vi "Inject Optitrack Position.vi"() -> (5 "Plug in titles":string[](array[string]), 7 "Plug in values":string[](array[string]))   [LabVIEW 2021]
uses:
  Controls/Post_Process.ctl
  Controls/Setup.ctl
  Globals/Meas_global.vi
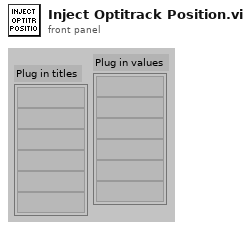
[diagram p1: front panel]
types:
  T1 = typedef "Setup.ctl" = enum16{"Run Program", "Show Setup", "Save Current Setup", "Setup Front Panel"}
  T2 = typedef "Post_Process.ctl" = enum16{"Take New Data", "Post Process Raw Data File"}
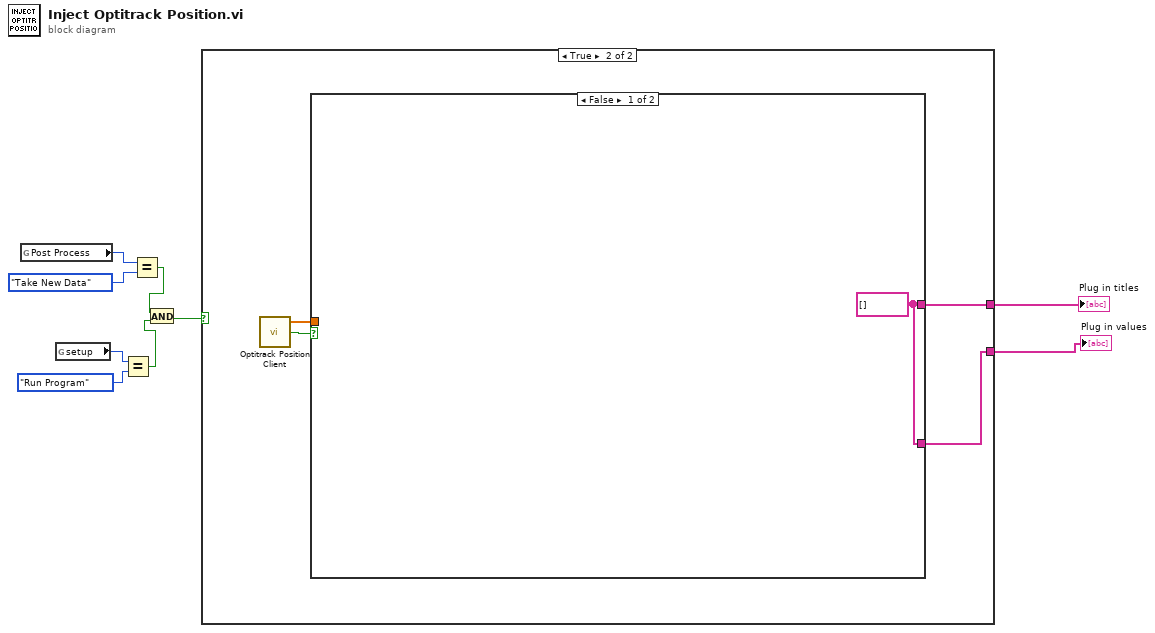
[diagram p0: block diagram]
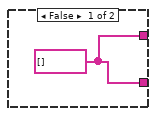
[diagram p2: hidden frame]
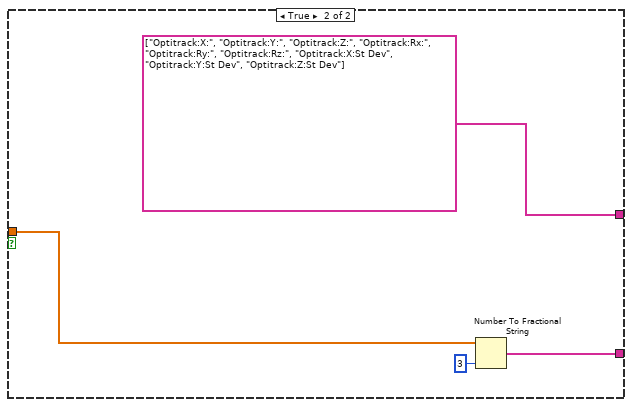
[diagram p3: hidden frame]
diagram:
  n1 = global read "Meas_global.vi" "Post Process"() -> (w4:T2)
  n2 = global read "Meas_global.vi" "setup"() -> (w6:T1)
  n3 = Equal?(x=w6, y=Setup."Run Program" ("setup")) -> (x = y?=w9:bool)
  n4 = Equal?(x=w4, y=Post_Process."Take New Data" ("Post Process")) -> (x = y?=w8:bool)
  n5 = And(x=w8, y=w9) -> (x .and. y?=w3:bool)
  n6 = case shown="True" w3 {
    tunnel: [w10 w14] -> w2
    tunnel: [w10 w12] -> w1
    frame False {
      w10 = string[] [] ("Plug in titles")
    }
    frame True {
      n7 = call "Optitrack Position Client.vi"() -> ("Position XYZ"=w13:dbl[], "Live?"=w11:bool)  [unwired: 2 in, 1 out]
      n8 = case shown="False" w11 {
        tunnel: [w15 string[] ["Optitrack:X:", "Optitrack:Y:", "Optitrack:Z:", "Optitrack:Rx:", "Optitrack:Ry:", "Optitrack:Rz:", "Optitrack:X:St Dev", "Optitrack:Y:St Dev", "Optitrack:Z:St Dev"] ("Plug in titles")] -> w14
        tunnel: w13 -> [_ w18]
        tunnel: [w15 w17] -> w12
        frame False {
          w15 = string[] [] ("Plug in titles")
        }
        frame True {
          n9 = Number To Fractional String(number=w18, precision (6)=i16 3) -> (F-format string=w17:string[])  [unwired: 2 in]
        }
      }
    }
  }
  "Plug in values" <- w1
  "Plug in titles" <- w2
